vi "importxml.vi"(7 "String":string, 10 "sc":string="/SC1") -> (0 "output array":T1(array[cluster])=[{[], "Voltage_cluster"={0.0, 0.0, 0.0, 0.0, TRUE, 0.0, 0.0}, "Strain_cluster"={0.0, 0.0, 0.0, 0.0, TRUE, 0.0, 0.0, 0.0, 0.0, ""}}, {[], "Voltage_cluster"={0.0, 0.0, 0.0, 0.0, TRUE, 0.0, 0.0}, "Strain_cluster"={0.0, 0.0, 0.0, 0.0, TRUE, 0.0, 0.0, 0.0, 0.0, ""}}, {[], "Voltage_cluster"={0.0, 0.0, 0.0, 0.0, TRUE, 0.0, 0.0}, "Strain_cluster"={0.0, 0.0, 0.0, 0.0, TRUE, 0.0, 0.0, 0.0, 0.0, ""}}, {[], "Voltage_cluster"={0.0, 0.0, 0.0, 0.0, TRUE, 0.0, 0.0}, "Strain_cluster"={0.0, 0.0, 0.0, 0.0, TRUE, 0.0, 0.0, 0.0, 0.0, ""}}, {[], "Voltage_cluster"={0.0, 0.0, 0.0, 0.0, TRUE, 0.0, 0.0}, "Strain_cluster"={0.0, 0.0, 0.0, 0.0, TRUE, 0.0, 0.0, 0.0, 0.0, ""}}, {[], "Voltage_cluster"={0.0, 0.0, 0.0, 0.0, TRUE, 0.0, 0.0}, "Strain_cluster"={0.0, 0.0, 0.0, 0.0, TRUE, 0.0, 0.0, 0.0, 0.0, ""}}, {[], "Voltage_cluster"={0.0, 0.0, 0.0, 0.0, TRUE, 0.0, 0.0}, "Strain_cluster"={0.0, 0.0, 0.0, 0.0, TRUE, 0.0, 0.0, 0.0, 0.0, ""}}, {[], "Voltage_cluster"={0.0, 0.0, 0.0, 0.0, TRUE, 0.0, 0.0}, "Strain_cluster"={0.0, 0.0, 0.0, 0.0, TRUE, 0.0, 0.0, 0.0, 0.0, ""}}])   [LabVIEW 2011]
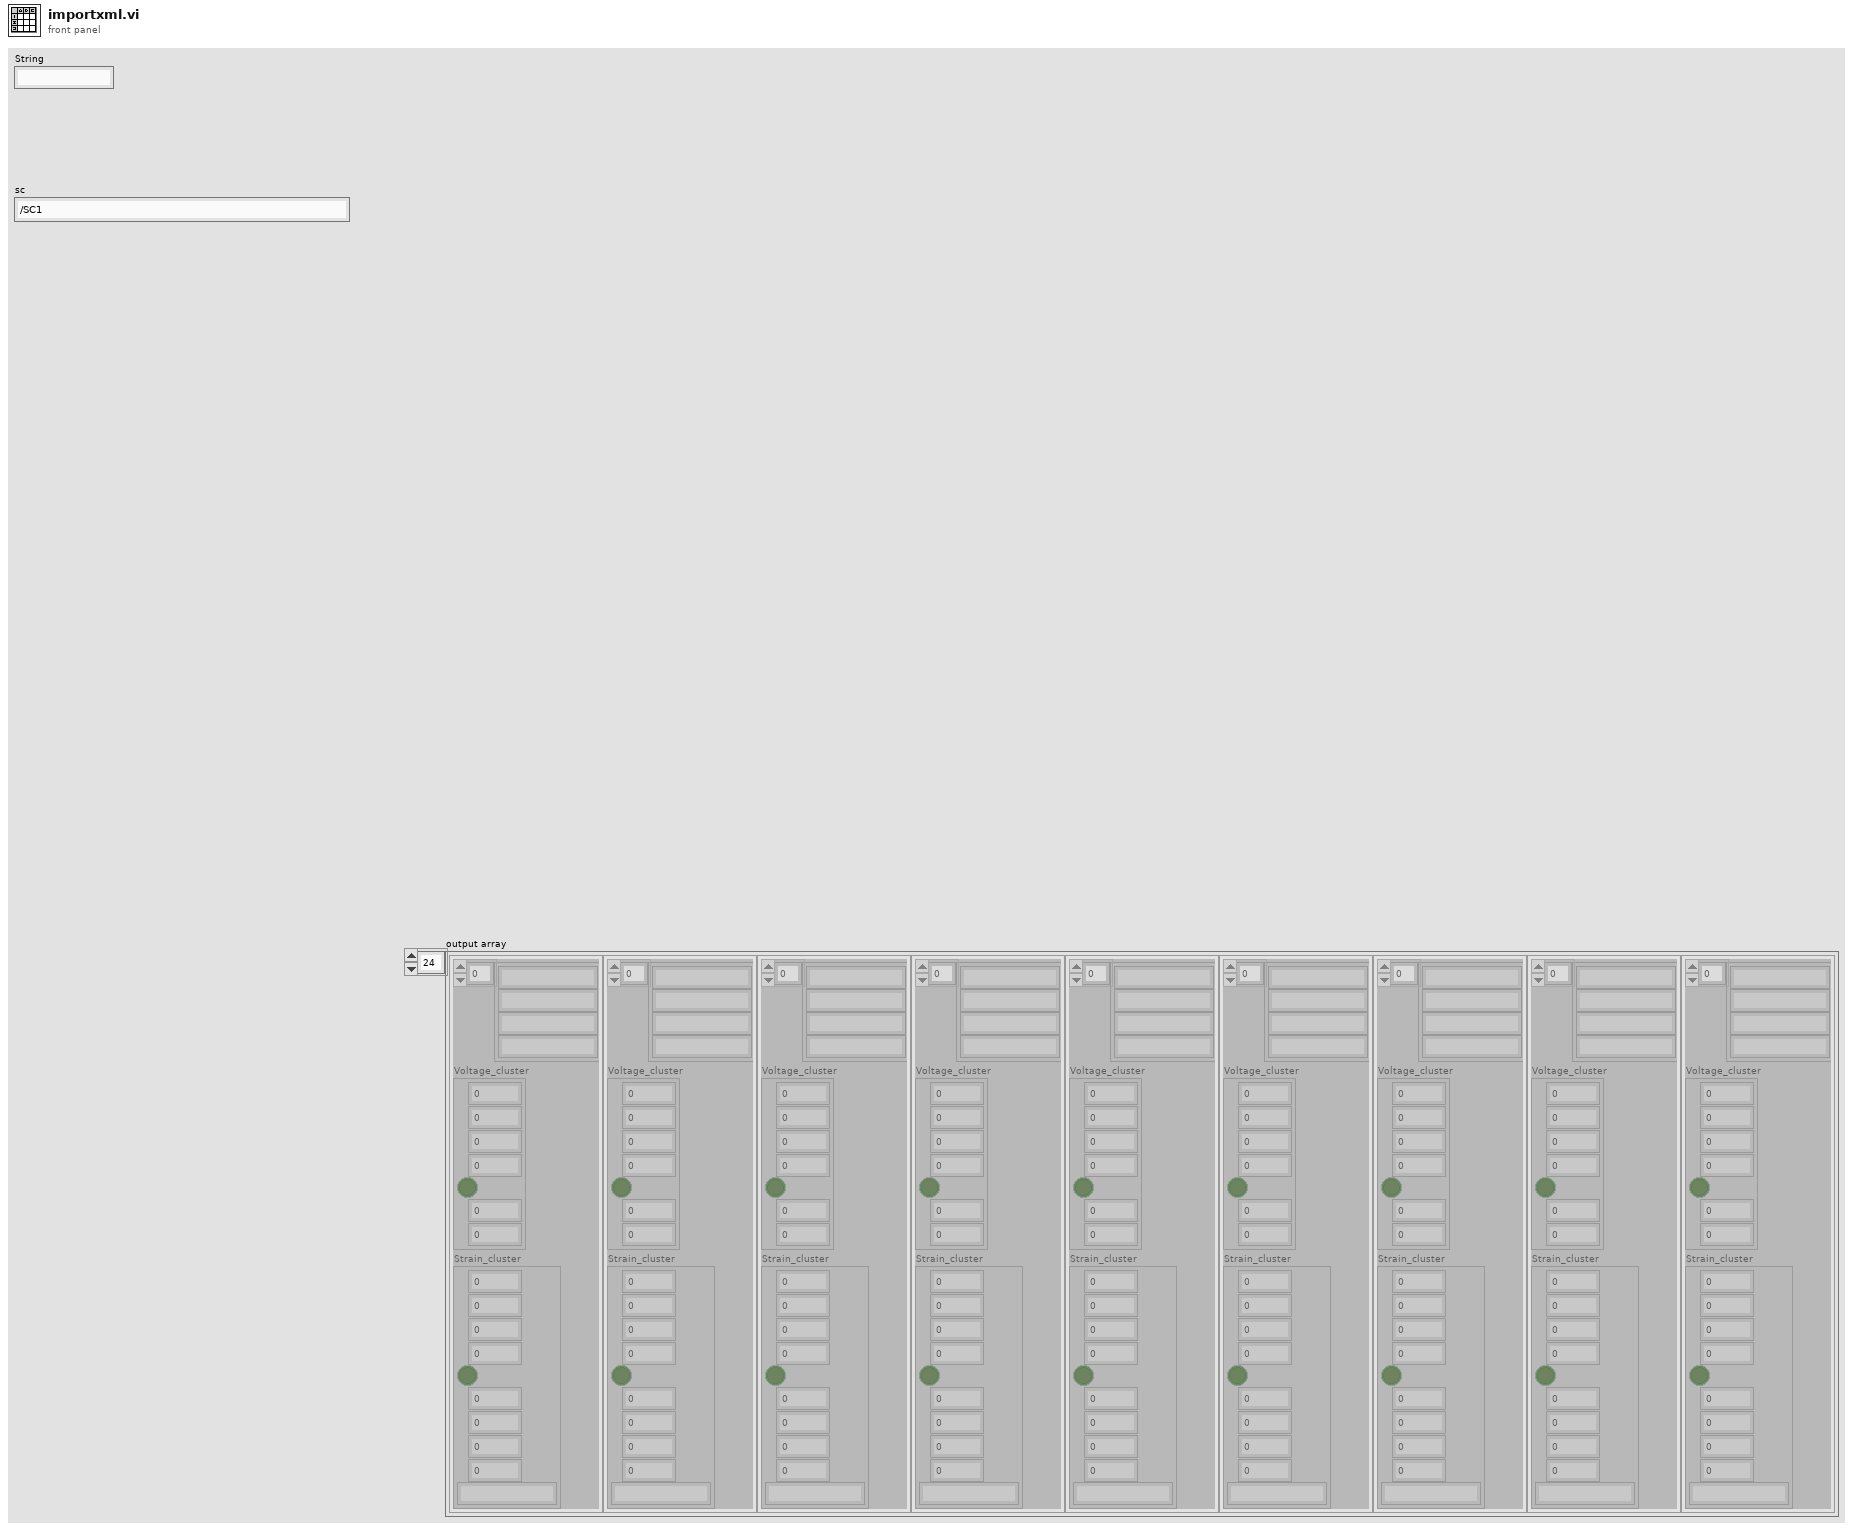
[diagram p1: front panel]
types:
  T1 = cluster{string[], "Voltage_cluster":cluster{dbl, dbl, dbl, dbl, bool, dbl, dbl}, "Strain_cluster":cluster{dbl, dbl, dbl, dbl, bool, dbl, dbl, dbl, dbl, string}}[]
  T2 = cluster{dbl, dbl, dbl, dbl, bool, dbl, dbl, dbl, dbl, string}
  T3 = cluster{string[], cluster{dbl, dbl, dbl, dbl, bool, dbl, dbl}, cluster{dbl, dbl, dbl, dbl, bool, dbl, dbl, dbl, dbl, string}}
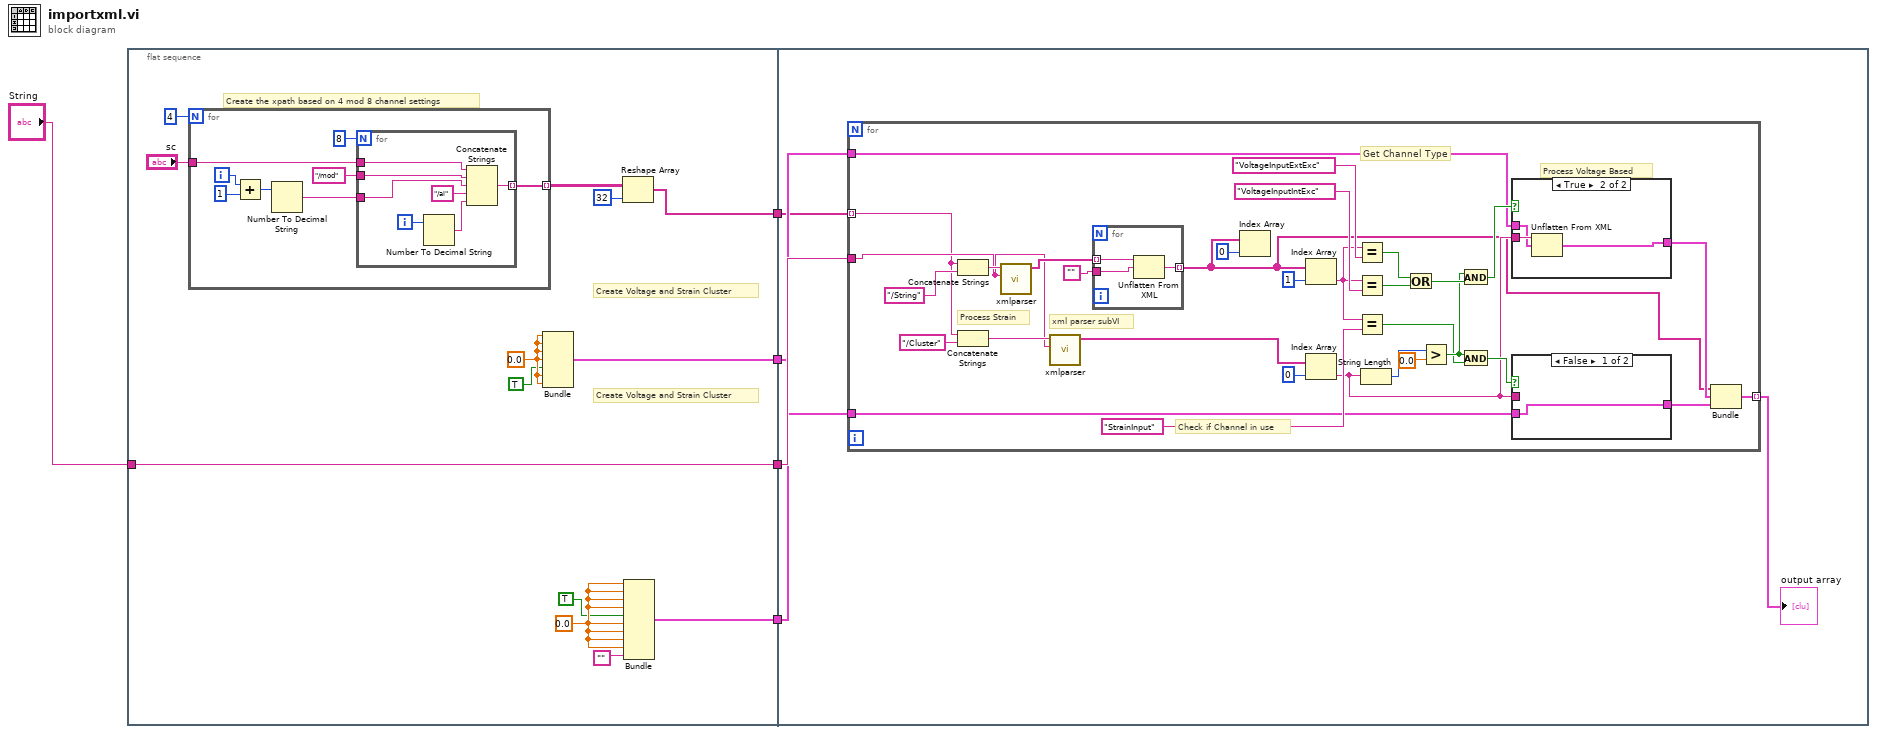
[diagram p0: block diagram]
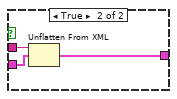
[diagram p2: hidden frame]
diagram:
  n1 = flat-sequence {
    tunnel: "String" -> [w9]
    tunnel: [w9] -> w4
    tunnel: [w8] -> w3
    tunnel: [w7] -> w2
    tunnel: [w6] -> w1
    tunnel: w4 -> [w38]
    tunnel: w3 -> [w37]
    tunnel: w2 -> [w36]
    tunnel: w1 -> [w35]
    frame #0 {
      w13 = 0.0
      w11 = 0.0
      # "Create Voltage and Strain Cluster"
      # "Create Voltage and Strain Cluster"
      # "Create the xpath based on 4 mod 8 channel settings"
      n2 = for {
        N: 4 -> [_]
        tunnel: [w23] -> w16 mode=indexing
        tunnel: "sc" -> [w26]
        i -> [w21]
        n3 = Add(x=w21, y=1) -> (x+y=w20:i32)
        n4 = Number To Decimal String(number=w20) -> (decimal integer string=w24:string)  [unwired: 1 in]
        n5 = for {
          N: 8 -> [_]
          tunnel: w26 -> [w33]
          tunnel: "/mod" -> [w32]
          tunnel: w24 -> [w31]
          tunnel: [w27] -> w23 mode=indexing
          i -> [w29]
          n6 = Number To Decimal String(number=w29) -> (decimal integer string=w28:string)  [unwired: 1 in]
          n7 = Concatenate Strings(w33, w32, w31, "/ai", w28) -> (w27:string)
        }
      }
      n8 = Bundle(w11, w11, w11, w11, TRUE, w11, w11) -> (w8:cluster{dbl, dbl, dbl, dbl, bool, dbl, dbl})  [unwired: 1 in]
      n9 = Reshape Array(w16, 32 ("dimension size")) -> (w6:string[])
      n10 = Bundle(w13, w13, w13, w13, TRUE, w13, w13, w13, w13, "") -> (w7:T2)  [unwired: 1 in]
    }
    frame #1 {
      n11 = for {
        tunnel: w38 -> [w40]
        tunnel: [w44] -> w34 mode=indexing
        tunnel: w37 -> [w42]
        tunnel: w36 -> [w41]
        tunnel: w35 -> [w39] mode=indexing
        # "Process Strain"
        # "Process Voltage Based"
        # "Check if Channel in use"
        # "Get Channel Type"
        # "xml parser subVI"
        n12 = Concatenate Strings(w39, "/String") -> (w63:string)
        n13 = Concatenate Strings(w39, "/Cluster") -> (w65:string)
        n14 = call "xmlparser.vi"("xml_file_content"=w40, "XPath expression"=w63) -> ("Array 2"=w51:string[])  [unwired: 9 in]
        n15 = call "xmlparser.vi"("xml_file_content"=w40, "XPath expression"=w65) -> ("Array 2"=w67:string[])  [unwired: 9 in]
        n16 = for {
          tunnel: w51 -> [w81] mode=indexing
          tunnel: "" -> [w80]
          tunnel: [w79] -> w43 mode=indexing
          n17 = Unflatten From XML(xml string=w81, type=w80) -> (value=w79:string)  [unwired: 1 in, 1 out]
        }
        n18 = Index Array(array=w43, index=0) -> ()  [unwired: 1 out]
        n19 = Index Array(array=w43, index=1) -> (element=w47:string)
        n20 = Index Array(array=w67, index=0) -> (element=w53:string)
        n21 = Equal?(x=w47, y="VoltageInputExtExc") -> (x = y?=w60:bool)
        n22 = Equal?(x=w47, y="VoltageInputIntExc") -> (x = y?=w59:bool)
        n23 = Equal?(x=w47, y="StrainInput") -> (x = y?=w55:bool)
        n24 = String Length(string=w53) -> (length=w70:i32)
        n25 = Or(x=w60, y=w59) -> (x .or. y?=w58:bool)
        n26 = Greater?(x=w70, y=0.0) -> (0:w56:bool)
        n27 = And(x=w56, y=w58) -> (x .and. y?=w52:bool)
        n28 = And(x=w56, y=w55) -> (x .and. y?=w54:bool)
        n29 = case shown="True" w52 {
          tunnel: w53 -> [_ w78]
          tunnel: [w75 w77] -> w46
          tunnel: w42 -> [w75 w76]
          frame False {
          }
          frame True {
            n30 = Unflatten From XML(xml string=w78, type=w76) -> (value=w77:cluster{dbl, dbl, dbl, dbl, bool, dbl, dbl})  [unwired: 1 in, 1 out]
          }
        }
        n31 = case shown="False" w54 {
          tunnel: w53 -> [_ w74]
          tunnel: [w71 w73] -> w45
          tunnel: w41 -> [w71 w72]
          frame False {
          }
          frame True {
            n32 = Unflatten From XML(xml string=w74, type=w72) -> (value=w73:T2)  [unwired: 1 in, 1 out]
          }
        }
        n33 = Bundle(w43, w46, w45) -> (w44:T3)  [unwired: 1 in]
      }
      "output array" <- w34
    }
  }
